vi "Teleop.vi"(10 "Match Info":T2={"Autonomous Elapsed Seconds"=0.0, "TeleOp Elapsed Seconds"=0.0, "Disabled Elapsed Seconds"=0.0, "Visited Autonomous"=FALSE, "Visited TeleOp"=FALSE, "Visited Disabled"=FALSE, "Autonomous Settings"={"Autonomous Style"=enum."Independent", "VI Refnum"=refnum}}, 11 "Call Context":T3) -> ()   [LabVIEW 2018]
doc: "This VI is called for each enabled TeleOp packet received from the DS. It is typically used to read from joysticks and other inputs and update I/O or setpoints for timed control loops. It should complete and return within 20 milliseconds or risk missing DS packets."
uses:
  <vilib>/Rock Robotics/WPI/DriverStation/WPI_DriverStationDerivedRobotMode.ctl
  <vilib>/Rock Robotics/WPI/DriverStation/WPI_DriverStationMatch Info.ctl
  <vilib>/Rock Robotics/WPI/Utilities/WPI_GetSetVariantRefNum.vi
  <vilib>/Rock Robotics/Network Tables/NT Write Boolean Array.vi
  <vilib>/Rock Robotics/Network Tables/NT Write Numeric Array.vi
  <vilib>/Rock Robotics/Network Tables/NT Write Boolean.vi
  <vilib>/Rock Robotics/Network Tables/NT Write Number.vi
  <vilib>/Rock Robotics/WPI/RobotDrive/WPI_RobotDriveMecanumDrive_Cartesian.vi
  <vilib>/Rock Robotics/WPI/ThirdParty/Phoenix-LabVIEW/Motor Controller/Get/CTRE_Phoenix_MotorController_GetSelectedSensorData.vi
  <vilib>/Rock Robotics/WPI/Ultrasonic/WPI_SonarSRF04DigitalRefNum Registry Get.vi
  <vilib>/Rock Robotics/WPI/Ultrasonic/WPI_SonarSRF04DigitalGetRange.vi
panel:
  out "YRPHfH":T1
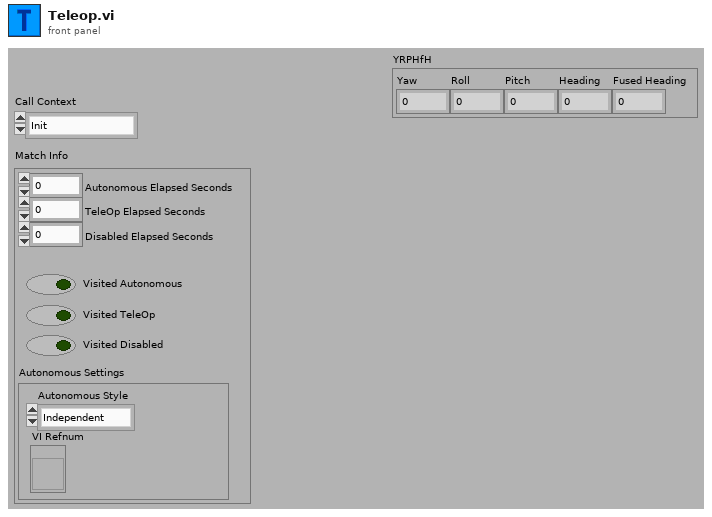
[diagram p1: front panel]
types:
  T1 = cluster{"Yaw":dbl, "Roll":dbl, "Pitch":dbl, "Heading":dbl, "Fused Heading":dbl}
  T2 = typedef "WPI_DriverStationMatch Info.ctl" = cluster{"Autonomous Elapsed Seconds":dbl, "TeleOp Elapsed Seconds":dbl, "Disabled Elapsed Seconds":dbl, "Visited Autonomous":bool, "Visited TeleOp":bool, "Visited Disabled":bool, "Autonomous Settings":cluster{"Autonomous Style":enum16{"Iterative", "Independent"}, "VI Refnum":refnum<vi>}}
  T3 = typedef "WPI_DriverStationDerivedRobotMode.ctl" = enum16{"Init", "Execute", "Stop"}
  T4 = typedef "WPI_JoystickDevRef.ctl" = cluster{"Device":T5}
  T5 = typedef "WPI_JoystickDeviceEnum.ctl" = enum16{"USB 0", "USB 1", "USB 2", "USB 3", "USB 4", "USB 5"}
  T6 = typedef "WPI_MotorControlDeviceRef.ctl" = cluster{"DeviceStatus":errorcluster, "Type":T7, "PWM":cluster{"PWM Channel":T8, "DeadBand":T9}, "CAN":cluster{"Device Number":u8, "SetOutput VI Ref":variant, "GetOutput VI Ref":variant, "Enable VI Ref":variant, "Disable VI Ref":variant, "Data":variant}, "Invert":bool, "DIO PWM":cluster{"PWM \"Enable\" Channel":T8, "DIOChannel":T10, "PWM Rate":dbl}}
  T7 = typedef "WPI_MotorControlType.ctl" = enum16{"PWM", "CAN", "DIO PWM"}
  T8 = typedef "FPGA_DIOPWMChannel.ctl" = enum8{"PWM 0", "PWM 1", "PWM 2", "PWM 3", "PWM 4", "PWM 5", "PWM 6", "PWM 7", "PWM 8", "PWM 9", "PWM MXP 0", "PWM MXP 1", "PWM MXP 2", "PWM MXP 3", "PWM MXP 4", "PWM MXP 5", "PWM MXP 6", "PWM MXP 7", "PWM MXP 8", "PWM MXP 9", "Invalid"}
  T9 = typedef "WPI_PWMDeadband.ctl" = cluster{"Name":string, "maxPositivePwm":i32, "minPositivePwm":i32, "centerPwm":i32, "maxNegativePwm":i32, "minNegativePwm":i32, "angularRange":u16}
  T10 = typedef "FPGA_DIOChannel.ctl" = enum8{"DIO 0", "DIO 1", "DIO 2", "DIO 3", "DIO 4", "DIO 5", "DIO 6", "DIO 7", "DIO 8", "DIO 9", "DIO MXP 0", "DIO MXP 1", "DIO MXP 2", "DIO MXP 3", "DIO MXP 4", "DIO MXP 5", "DIO MXP 6", "DIO MXP 7", "DIO MXP 8", "DIO MXP 9", "DIO MXP 10", "DIO MXP 11", "DIO MXP 12", "DIO MXP 13", "DIO MXP 14", "DIO MXP 15", "SPI Port CS1", "SPI Port CS2", "SPI Port CS3", "SPI Port MISO", "SPI Port MOSI", "Invalid"}
  T11 = typedef "WPI_RobotDriveDevRef.ctl" = cluster{"DevStatus":errorcluster, "Motors[]":T6[], "Square Inputs":bool, "Max Output":dbl}
  T12 = typedef "Command Status Info.ctl" = cluster{"Name":string, "Status":T13, "notifier out":T14}
  T13 = typedef "Completion Status.ctl" = enum16{"Successful", "Aborted", "Incomplete"}
  T14 = typedef "Completion Notifier.ctl" = refnum<notifier>
  T15 = typedef "WPI_UltrasonicDeviceRef.ctl" = cluster{"DevStatus":errorcluster, "Ping Channel":T10, "Echo Channel":T10, "CntIndex":T16}
  T16 = typedef "FPGA_CounterCtrSystemIndex.ctl" = enum8{"Ctr 0", "Ctr 1", "Ctr 2", "Ctr 3", "Ctr 4", "Ctr 5", "Ctr 6", "Ctr 7", "Invalid"}
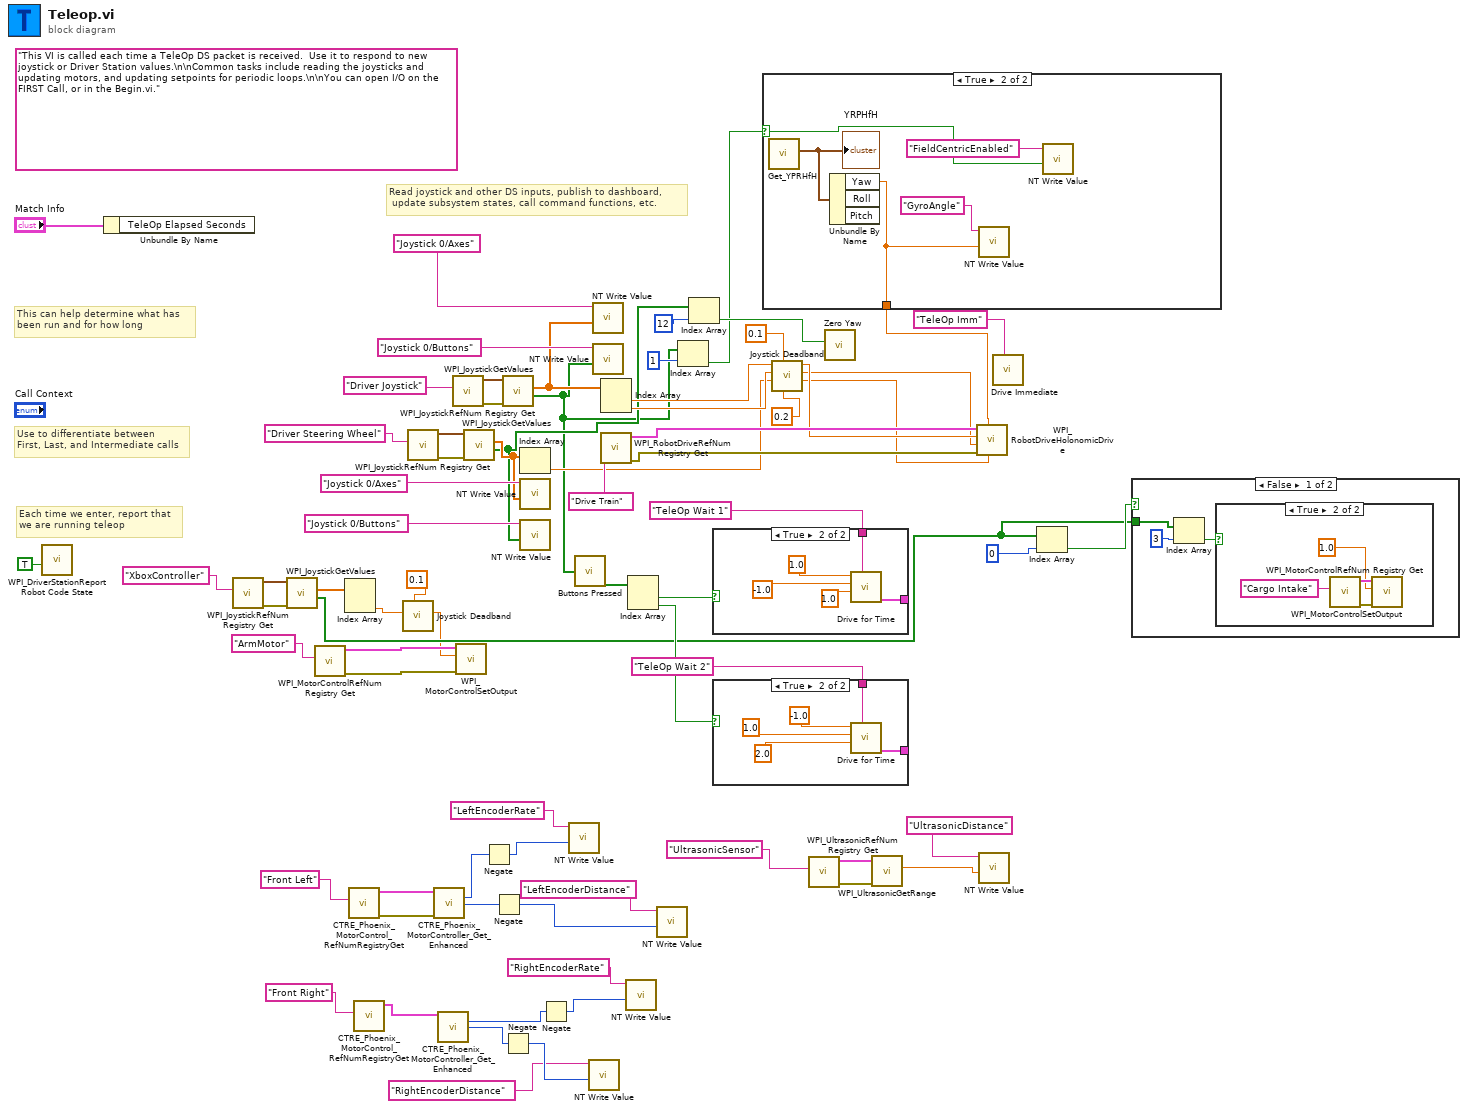
[diagram p0: block diagram]
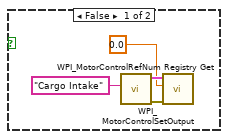
[diagram p2: hidden frame]
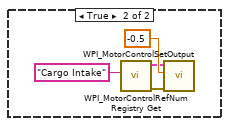
[diagram p3: hidden frame]
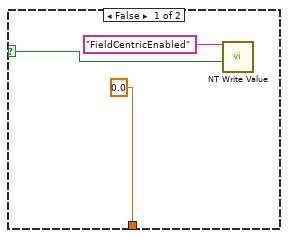
[diagram p4: hidden frame]
diagram:
  (unwired) "This VI is called each time a TeleOp DS packet is received.  Use it to respond to new joystick or Driver Station values.\n\nCommon tasks include reading the joysticks and updating motors, and updating setpoints for periodic loops.\n\nYou can open I/O on the FIRST Call, or in the Begin.vi."
  # "Read joystick and other DS inputs, publish to dashboard,\n update subsystem states, call command functions, etc."
  # "Each time we enter, report that\nwe are running teleop"
  # "Use to differentiate between\nFirst, Last, and Intermediate calls"
  # "This can help determine what has\nbeen run and for how long"
  n1 = call <vilib>:"WPI_DriverStationReport Robot Code State.vi"("TeleOp"=TRUE ("Autonomous")) -> ()  [unwired: 10 in, 1 out]
  n2 = Unbundle By Name("Match Info") -> ()  [unwired: 1 out]
  n3 = call <vilib>:"WPI_JoystickRefNum Registry Get.vi"("refnum name"="XboxController") -> ("error out"=w11:errorcluster, "JoystickDevRef"=w10:T4)  [unwired: 9 in]
  n4 = call <vilib>:"WPI_JoystickGetValues.vi"("error in (no error)"=w11, "JoystickDevRef"=w10) -> ("Buttons"=w4:bool[], "Axes"=w6:dbl[])  [unwired: 5 in, 3 out]
  n5 = call <vilib>:"WPI_MotorControlRefNum Registry Get.vi"("refnum name"="ArmMotor") -> ("error out"=w8:errorcluster, "MotorControlDevRef"=w7:T6)  [unwired: 9 in]
  n6 = Index Array(array=w6) -> (element #2=w3:dbl)  [unwired: 2 in, 1 out]
  n7 = call <vilib>:"CTRE_Phoenix_MotorControl_RefNumRegistryGet.vi"("refnum name"="Front Left") -> ("error out"=w32:errorcluster, "PhoenixMotorControlDevRef"=w33:T6)  [unwired: 9 in]
  n8 = call <vilib>:"CTRE_Phoenix_MotorControl_RefNumRegistryGet.vi"("refnum name"="Front Right") -> ("PhoenixMotorControlDevRef"=w29:T6)  [unwired: 9 in, 1 out]
  n9 = call "Joystick Deadband.vi"("X Y Deadband"=0.1, "Y"=w3) -> ("Y Out"=w1:dbl)  [unwired: 7 in, 2 out]
  n10 = call <vilib>:"WPI_JoystickRefNum Registry Get.vi"("refnum name"="Driver Steering Wheel") -> ("error out"=w59:errorcluster, "JoystickDevRef"=w58:T4)  [unwired: 9 in]
  n11 = call-poly <vilib>:"CTRE_Phoenix_MotorController_Get_Enhanced.vi"("PhoenixMotorControlDevRef"=w33, "error in"=w32) -> ("Position (Raw Sensor Units)"=w31:i32, "Velocity (Raw Sensor Units per 100 ms)"=w21:i32)  [unwired: 10 in, 2 out]
  n12 = call-poly <vilib>:"CTRE_Phoenix_MotorController_Get_Enhanced.vi"("PhoenixMotorControlDevRef"=w29) -> ("Position (Raw Sensor Units)"=w25:i32, "Velocity (Raw Sensor Units per 100 ms)"=w24:i32)  [unwired: 11 in, 2 out]
  n13 = call <vilib>:"WPI_JoystickRefNum Registry Get.vi"("refnum name"="Driver Joystick") -> ("error out"=w57:errorcluster, "JoystickDevRef"=w70:T4)  [unwired: 1 in, 8 out]
  n14 = call <vilib>:"WPI_MotorControlSetOutput.vi"("error in (no error)"=w8, "Output"=w1, "MotorControlDevRef"=w7) -> ()  [unwired: 6 in, 3 out]
  n15 = call <vilib>:"WPI_JoystickGetValues.vi"("error in (no error)"=w59, "JoystickDevRef"=w58) -> ("Buttons"=w41:bool[], "Axes"=w54:dbl[])  [unwired: 5 in, 3 out]
  n16 = Negate(x=w31) -> (-x=w30:i32)
  n17 = Negate(x=w21) -> (-x=w22:i32)
  n18 = call <vilib>:"WPI_JoystickGetValues.vi"("error in (no error)"=w57, "JoystickDevRef"=w70) -> ("Buttons"=w13:bool[], "Axes"=w62:dbl[])  [unwired: 5 in, 3 out]
  n19 = Negate(x=w24) -> (-x=w26:i32)
  n20 = Index Array(array=w54) -> (element=w46:dbl)  [unwired: 1 in]
  n21 = call-poly <vilib>:"NT Write Value.vi"("Numeric Array"=w54, "Name"="Joystick 0/Axes") -> ()  [unwired: 9 in, 1 out]
  n22 = call-poly <vilib>:"NT Write Value.vi"("Boolean Array"=w41, "Name"="Joystick 0/Buttons") -> ()  [unwired: 9 in, 1 out]
  n23 = Negate(x=w25) -> (-x=w27:i32)
  n24 = call-poly <vilib>:"NT Write Value.vi"("Numeric"=w30, "Name"="LeftEncoderRate") -> ()  [unwired: 9 in, 1 out]
  n25 = call "Buttons Pressed.vi"("Button Values"=w13) -> ("Button Presses"=w66:bool[])
  n26 = call-poly <vilib>:"NT Write Value.vi"("Numeric"=w26, "Name"="RightEncoderDistance") -> ()  [unwired: 9 in, 1 out]
  n27 = call-poly <vilib>:"NT Write Value.vi"("Numeric Array"=w62, "Name"="Joystick 0/Axes") -> ()  [unwired: 9 in, 1 out]
  n28 = call-poly <vilib>:"NT Write Value.vi"("Boolean Array"=w13, "Name"="Joystick 0/Buttons") -> ()  [unwired: 9 in, 1 out]
  n29 = Index Array(array=w62) -> (element #1=w50:dbl, element #2=w48:dbl)  [unwired: 2 in]
  n30 = call <vilib>:"WPI_RobotDriveRefNum Registry Get.vi"("refnum name"="Drive Train") -> ("error out"=w53:errorcluster, "RobotDriveDevRef"=w52:T11)  [unwired: 9 in]
  n31 = call-poly <vilib>:"NT Write Value.vi"("Numeric"=w27, "Name"="RightEncoderRate") -> ()  [unwired: 9 in, 1 out]
  n32 = Index Array(array=w66) -> (element #1=w65:bool, element #2=w64:bool)  [unwired: 2 in]
  n33 = call-poly <vilib>:"NT Write Value.vi"("Numeric"=w22, "Name"="LeftEncoderDistance") -> ()  [unwired: 9 in, 1 out]
  n34 = Index Array(array=w13, index=1) -> (element=w37:bool)
  n35 = Index Array(array=w41, index=12) -> (element=w40:bool)
  n36 = case shown="True" w65 {
    tunnel: [_ w77] -> _
    tunnel: "TeleOp Wait 1" ("Description") -> [_ w76]
    frame False {
    }
    frame True {
      n37 = call "Drive for Time.vi"("Description"=w76, "Seconds"=1.0, "Right Speed"=-1.0, "Left Speed"=1.0) -> ("Command Info Out"=w77:T12)  [unwired: 6 in, 1 out]
    }
  }
  n38 = case shown="True" w64 {
    tunnel: [_ w81] -> _
    tunnel: "TeleOp Wait 2" ("Description") -> [_ w80]
    frame False {
    }
    frame True {
      n39 = call "Drive for Time.vi"("Description"=w80, "Seconds"=2.0, "Right Speed"=1.0, "Left Speed"=-1.0) -> ("Command Info Out"=w81:T12)  [unwired: 6 in, 1 out]
    }
  }
  n40 = case shown="True" w37 {
    selector: w37 -> [w84 w90]
    tunnel: [0.0 w87] -> w38
    frame False {
      n41 = call-poly <vilib>:"NT Write Value.vi"("Boolean"=w84, "Name"="FieldCentricEnabled") -> ()  [unwired: 9 in, 1 out]
    }
    frame True {
      n42 = call <vilib>:"Get_YPRHfH.vi"() -> ("YRPHfH"=w91:T1)  [unwired: 11 in]
      "YRPHfH" <- w91
      n43 = Unbundle By Name(w91) -> ("Yaw"=w87:dbl)  [unwired: 2 out]
      n44 = call-poly <vilib>:"NT Write Value.vi"("Numeric"=w87, "Name"="GyroAngle") -> ()  [unwired: 9 in, 1 out]
      n45 = call-poly <vilib>:"NT Write Value.vi"("Boolean"=w90, "Name"="FieldCentricEnabled") -> ()  [unwired: 9 in, 1 out]
    }
  }
  n46 = call "Joystick Deadband.vi"("Z Deadband"=0.2, "X Y Deadband"=0.1, "Z"=w46, "Y"=w48, "X"=w50) -> ("Z Out"=w45:dbl, "Y Out"=w47:dbl, "X Out"=w49:dbl)  [unwired: 4 in]
  n47 = call-poly <vilib>:"WPI_UltrasonicRefNum Registry Get.vi"("refnum name"="UltrasonicSensor") -> ("error out"=w17:errorcluster, "SonarSRF04DevRef"=w18:T15)  [unwired: 9 in]
  n48 = call <vilib>:"Zero Yaw.vi"("Zero"=w40) -> ()  [unwired: 11 in]
  n49 = call-poly <vilib>:"WPI_UltrasonicGetRange.vi"("error in (no error)"=w17, "SonarSRF04DevRef"=w18) -> ("Distance"=w16:dbl)  [unwired: 7 in, 2 out]
  n50 = call-poly <vilib>:"WPI_RobotDriveHolonomicDrive.vi"("Rotation"=w45, "Gyro Angle"=w38, "error in (no error)"=w53, "Y"=w47, "X"=w49, "RobotDriveDevRef"=w52) -> ()  [unwired: 3 in, 3 out]
  n51 = call-poly <vilib>:"NT Write Value.vi"("Numeric"=w16, "Name"="UltrasonicDistance") -> ()  [unwired: 9 in, 1 out]
  n52 = call "Drive Immediate.vi"("Description"="TeleOp Imm") -> ()  [unwired: 10 in, 1 out]
  n53 = Index Array(array=w4, index=0) -> (element=w5:bool)
  n54 = case shown="False" w5 {
    tunnel: w4 -> [w93 _]
    frame False {
      n55 = Index Array(array=w93, index=3) -> (element=w92:bool)
      n56 = case shown="True" w92 {
        frame False {
          n57 = call <vilib>:"WPI_MotorControlRefNum Registry Get.vi"("refnum name"="Cargo Intake") -> ("error out"=w98:errorcluster, "MotorControlDevRef"=w97:T6)  [unwired: 9 in]
          n58 = call <vilib>:"WPI_MotorControlSetOutput.vi"("error in (no error)"=w98, "Output"=0.0, "MotorControlDevRef"=w97) -> ()  [unwired: 6 in, 3 out]
        }
        frame True {
          n59 = call <vilib>:"WPI_MotorControlRefNum Registry Get.vi"("refnum name"="Cargo Intake") -> ("error out"=w100:errorcluster, "MotorControlDevRef"=w101:T6)  [unwired: 9 in]
          n60 = call <vilib>:"WPI_MotorControlSetOutput.vi"("error in (no error)"=w100, "Output"=1.0, "MotorControlDevRef"=w101) -> ()  [unwired: 6 in, 3 out]
        }
      }
    }
    frame True {
      n61 = call <vilib>:"WPI_MotorControlRefNum Registry Get.vi"("refnum name"="Cargo Intake") -> ("error out"=w103:errorcluster, "MotorControlDevRef"=w104:T6)  [unwired: 9 in]
      n62 = call <vilib>:"WPI_MotorControlSetOutput.vi"("error in (no error)"=w103, "Output"=-0.5, "MotorControlDevRef"=w104) -> ()  [unwired: 6 in, 3 out]
    }
  }
